vi "Function.vi"(8 "error in (no error)":errorcluster, 10 "String A":string, 11 "One Terminal in":refnum<class "ToLower_STR.lvclass">) -> (0 "error out":errorcluster, 2 "String":string, 3 "One Terminal out":refnum<class "ToLower_STR.lvclass">)   [LabVIEW 2021, in "ToLower_STR.lvclass"]
uses:
  ToLower_STR.lvclass
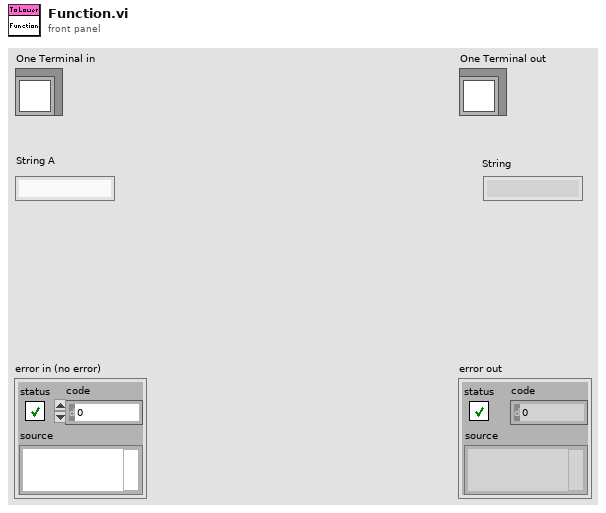
[diagram p1: front panel]
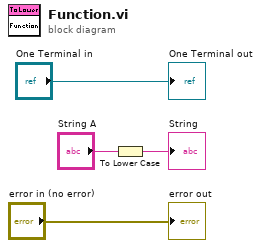
[diagram p0: block diagram]
diagram:
  n1 = To Lower Case(string="String A") -> (all lower case string=→"String":string)
  "error out" <- "error in (no error)"
  "One Terminal out" <- "One Terminal in"
